vi "test Import Major and Minor Frames.vi"(8 "error in":errorcluster, 11 "TestCase in":refnum<class "1553 Parameters Import.lvclass">) -> (0 "error out":errorcluster, 3 "TestCase out":refnum<class "1553 Parameters Import.lvclass">)   [LabVIEW 2020, in "1553 Parameters Import.lvclass"]
uses:
  1553 Parameters Import.lvclass
  <vilib>/addons/_JKI Toolkits/VI Tester/TestCase.llb/TestCase.lvclass
  Shared/Major Frame Definition.ctl
  Shared/Minor Frame Definition.ctl
  C:/Program Files (x86)/National Instruments/LabVIEW 2020/vi.lib/addons/_JKI Toolkits/VI Tester/TestCase.llb/TestCase.lvclass
  C:/dev/git/niveristand-aim-milStd1553-custom-device/Source/Custom Device Support/Tests/Unit/Import/1553 Parameters Import.lvclass
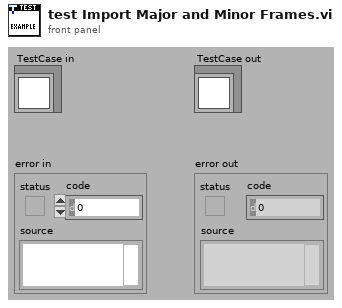
[diagram p1: front panel]
types:
  T1 = typedef "Minor Frame Definition.ctl" = cluster{"name":string, "messages":string[]}
  T2 = typedef "Major Frame Definition.ctl" = cluster{"name":string, "minor frames":string[]}
  T3 = typedef "BIU Configuration.ctl" = cluster{"HW channel":u16, "terminal addresses":T4[], "terminal names":string[], "major frames":T2[], "minor frames":T1[], "acyclic frames":T5[], "messages":T6[], "minor frame period (us)":i32}
  T4 = typedef "Address.ctl" = u16
  T5 = typedef "Acyclic Frame Definition.ctl" = cluster{"name":string, "messages":string[]}
  T6 = typedef "Message Definition.ctl" = cluster{"name":string, "message type":T7, "endpoint Tx":T8, "endpoint Rx":T8, "create timestamp channel":bool, "mode code":u16, "number of words":u16, "parameters":cluster{"name":string, "default value":dbl, "unit":string, "parameter definition":T9}[]}
  T7 = typedef "Message Type.ctl" = string
  T8 = typedef "Terminal Endpoint.ctl" = cluster{"terminal address":T4, "subaddress":T4}
  T9 = typedef "Parameter Definition.ctl" = cluster{"start index":i32, "size (bits)":i32, "encoding":enum16{"BNR", "BCD", "Discrete"}, "signed":bool, "multiplier":dbl, "offset":dbl}
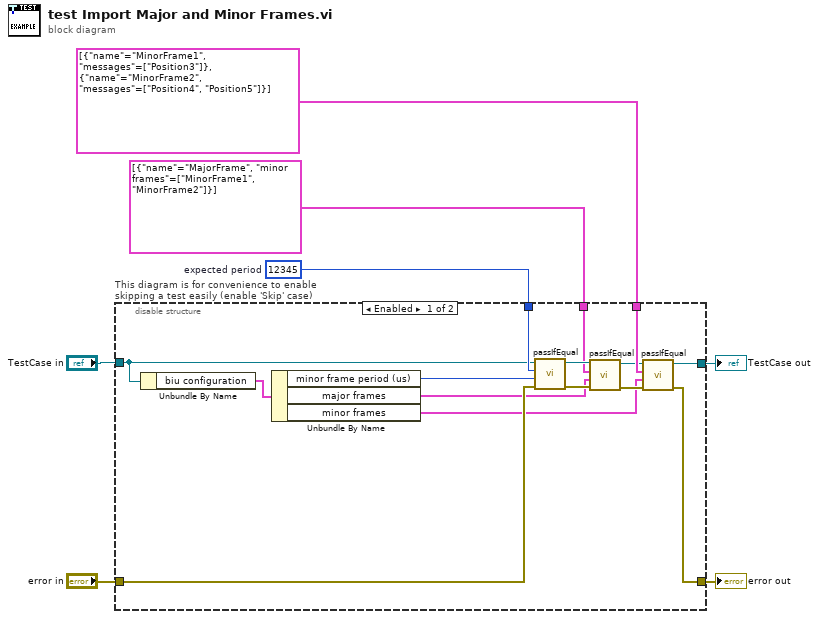
[diagram p0: block diagram]
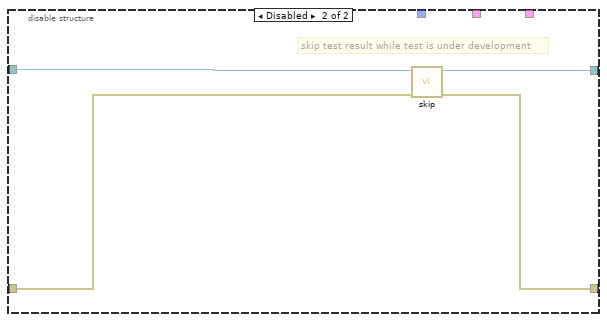
[diagram p2: hidden frame]
diagram:
  w3 = 12345  # expected period
  n1 = disable-structure "This diagram is for convenience to enable skipping a test easily (enable 'Skip' case)" shown="Enabled" {
    disable-tunnel: "TestCase in" -> [w8 w26]
    disable-tunnel: [w21 w24] -> w4
    disable-tunnel: [w20 w25] -> w6
    disable-tunnel: "error in" -> [w19 w23]
    disable-tunnel: w3 -> [w14 _]
    disable-tunnel: T2[] [{"name"="MajorFrame", "minor frames"=["MinorFrame1", "MinorFrame2"]}] ("major frames") -> [w12 _]
    disable-tunnel: T1[] [{"name"="MinorFrame1", "messages"=["Position3"]}, {"name"="MinorFrame2", "messages"=["Position4", "Position5"]}] ("minor frames") -> [w10 _]
    frame Enabled {
      n2 = Unbundle By Name(w8) -> ("biu configuration"=w22:T3)
      n3 = Unbundle By Name(w22) -> ("minor frame period (us)"=w15:i32, "major frames"=w13:T2[], "minor frames"=w11:T1[])
      n4 = call-dynamic "passIfEqual.vi"("error in (no error)"=w19, "y"=w15, "x"=w14, "TestCase in"=w8) -> ("error out"=w18:errorcluster, "TestCase out"=w17:refnum<class "1553 Parameters Import.lvclass">)  [unwired: 6 in]
      n5 = call-dynamic "passIfEqual.vi"("error in (no error)"=w18, "y"=w13, "x"=w12, "TestCase in"=w17) -> ("error out"=w16:errorcluster, "TestCase out"=w9:refnum<class "1553 Parameters Import.lvclass">)  [unwired: 6 in]
      n6 = call-dynamic "passIfEqual.vi"("error in (no error)"=w16, "y"=w11, "x"=w10, "TestCase in"=w9) -> ("error out"=w20:errorcluster, "TestCase out"=w21:refnum<class "1553 Parameters Import.lvclass">)  [unwired: 6 in]
    }
    frame Disabled {
      # "skip test result while test is under development"
      n7 = call <vilib>:"skip.vi"("error in (no error)"=w23, "TestCase in"=w26) -> ("error out"=w25:errorcluster, "TestCase out"=w24:refnum<class "1553 Parameters Import.lvclass">)  [unwired: 8 in]
    }
  }
  "error out" <- w6
  "TestCase out" <- w4
